vi "CheckSelectionStability.vi"() -> ()   [LabVIEW 2016]
uses:
  MFCdescription.ctl
  MFCcapability.ctl
panel:
  in  "currentCombo":T1[](array[typedef])
  in  "MFCcapabilities":T1[](array[typedef])
  in  "Max":dbl=350.0 format="%#_13g"
  in  "Increment":dbl=1.0
  out "XY Graph":cluster{dbl[], dbl[]}[](graph)
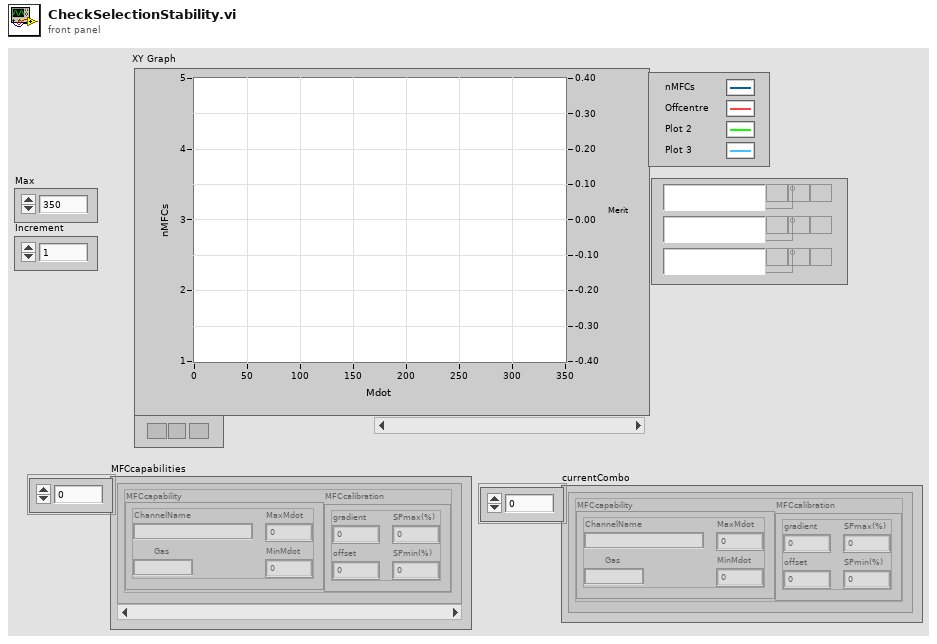
[diagram p1: front panel]
types:
  T1 = typedef "MFCdescription.ctl" = cluster{"MFCcapability":T2, "MFCcalibration":cluster{"gradient":dbl, "offset":dbl, "SPmin(%)":dbl, "SPmax(%)":dbl}}
  T2 = typedef "MFCcapability.ctl" = cluster{"ChannelName":string, "MinMdot":dbl, "MaxMdot":dbl, "Gas":string}
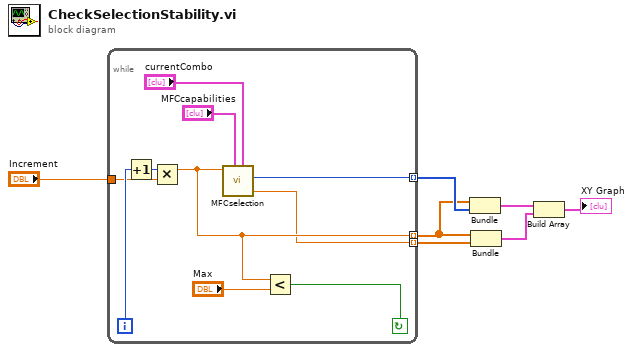
[diagram p0: block diagram]
diagram:
  n1 = while {
    tunnel: [w17] -> w7 mode=indexing
    tunnel: [w14] -> w4 mode=indexing
    tunnel: "Increment" -> [w15]
    tunnel: [w11] -> w3 mode=indexing
    i -> [w16]
    stop <- w12 continue-if-true
    n2 = Increment(x=w16) -> (x+1=w10:i32)
    n3 = Multiply(x=w10, y=w15) -> (x*y=w14:dbl)
    n4 = call "MFCselection.vi"("currentCombo"="currentCombo", "MFCcapabilities"="MFCcapabilities", "Mdot"=w14) -> ("Merit"=w11:dbl, "nMFCs"=w17:i32)  [unwired: 4 in, 1 out]
    n5 = Less?(x=w14, y="Max") -> (x < y?=w12:bool)
  }
  n6 = Bundle(w4, w7) -> (w6:cluster{dbl[], i32[]})  [unwired: 1 in]
  n7 = Bundle(w4, w3) -> (w1:cluster{dbl[], dbl[]})  [unwired: 1 in]
  n8 = Build Array(w6, w1) -> (→"XY Graph":cluster{dbl[], dbl[]}[])
